vi "AB Collect Samples.vi"(7 "Number Of Samples":i32, 9 "LBCB Number":T1, 10 "Reading In":dbl[](array[numeric]), 11 "Start":bool) -> (1 "Samples":i32, 2 "Average":dbl[](array[numeric]), 4 "Done":bool)   [LabVIEW 2013]
uses:
  Data Access Objects/Metadata/LBCB Number.ctl
  LBCB Data Accumulator.ctl
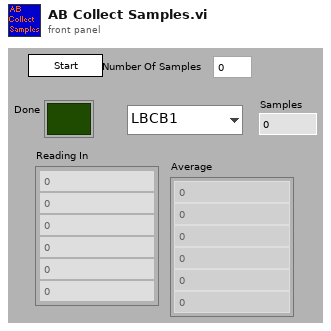
[diagram p1: front panel]
types:
  T1 = typedef "LBCB Number.ctl" = enum16{"LBCB1", "LBCB2"}
  T2 = typedef "LBCB Data Accumulator.ctl" = cluster{"Accum":dbl[], "Total":i32}
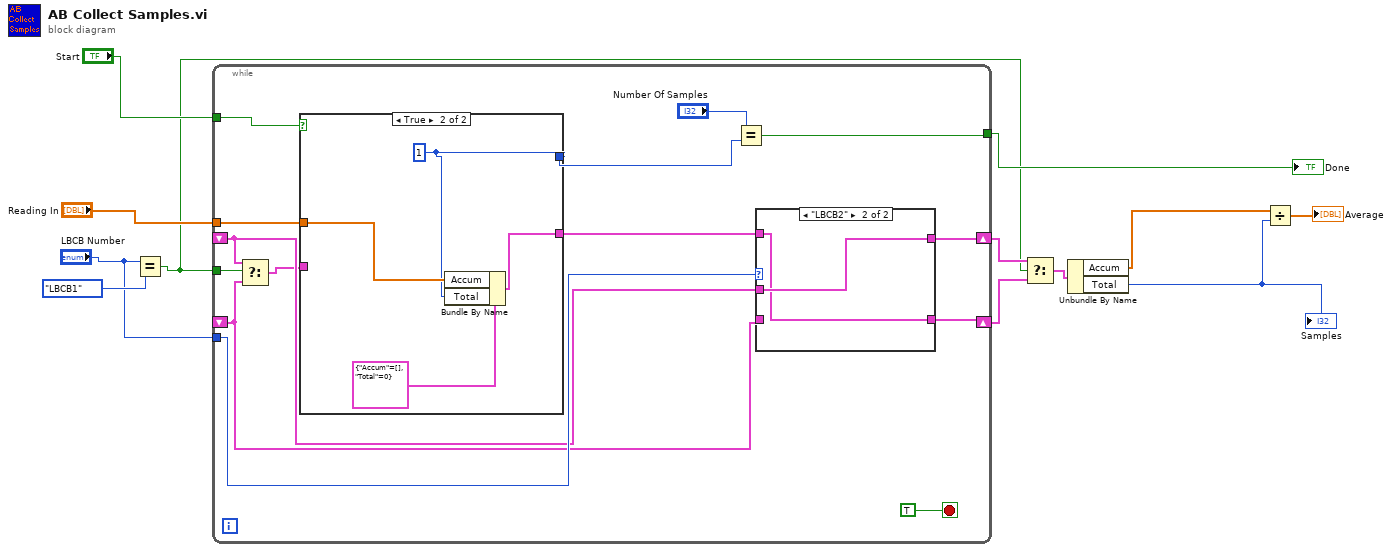
[diagram p0: block diagram]
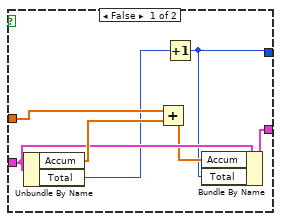
[diagram p3: hidden frame]
diagram:
  n1 = Equal?(x="LBCB Number", y=LBCB_Number."LBCB1") -> (x = y?=w5:bool)
  n2 = while {
    shift-right: [w15] -> w7
    shift-left: _ -> [w17]
    tunnel: "Start" -> [w25]
    tunnel: "Reading In" -> [w24]
    tunnel: [w21] -> w10
    shift-right: [w14] -> w6
    shift-left: _ -> [w16]
    tunnel: w5 -> [w20]
    tunnel: "LBCB Number" -> [w19]
    stop <- TRUE stop-if-true
    n3 = Select(t=w17, s=w20, f=w16) -> (s? t:f=w13:T2)
    n4 = case shown="True" w25 {
      tunnel: [w32 w39] -> w22
      tunnel: w24 -> [w37 w40]
      tunnel: [w31 w38] -> w18
      tunnel: w13 -> [w35 _]
      frame False {
        n5 = Unbundle By Name(w35) -> ("Accum"=w36:dbl[], "Total"=w33:i32)
        n6 = Add(x=w37, y=w36) -> (x+y=w34:dbl[])
        n7 = Increment(x=w33) -> (x+1=w32:i32)
        n8 = Bundle By Name(cluster=w35, "Accum"=w34, "Total"=w32) -> (w31:T2)
      }
      frame True {
        w39 = 1
        n9 = Bundle By Name(cluster=T2 {"Accum"=[], "Total"=0} ("LBCB Data Accum"), "Accum"=w40, "Total"=w39) -> (w38:T2)
      }
    }
    n10 = Equal?(x="Number Of Samples", y=w22) -> (x = y?=w21:bool)
    n11 = case shown="\"LBCB2\"" w19 {
      tunnel: w18 -> [w28 w29]
      tunnel: w17 -> [_ w30]
      tunnel: w16 -> [w27 _]
      tunnel: [w28 w30] -> w15
      tunnel: [w27 w29] -> w14
      frame "LBCB1" {
      }
      frame "LBCB2" {
      }
    }
  }
  "Done" <- w10
  n12 = Select(t=w7, s=w5, f=w6) -> (s? t:f=w4:T2)
  n13 = Unbundle By Name(w4) -> ("Accum"=w3:dbl[], "Total"=w2:i32)
  "Samples" <- w2
  n14 = Divide(x=w3, y=w2) -> (x/y=→"Average":dbl[])
